vi "Init Device.vi"(8 "error in (no error)":errorcluster, 11 "TE2000 in":refnum<class "Eclipse TI.lvclass">) -> (0 "error out":errorcluster, 3 "TE2000 out":refnum<class "Eclipse TI.lvclass">)   [LabVIEW 2015, in "Eclipse TI.lvlib" / "Eclipse TI.lvclass"]
uses:
  Eclipse TI.lvclass
  Eclipse TI.lvclass/Eclipse TI.ctl
  <vilib>/Instr/_visa.llb/VISA Configure Serial Port (Instr).vi
  Device/Device.lvclass
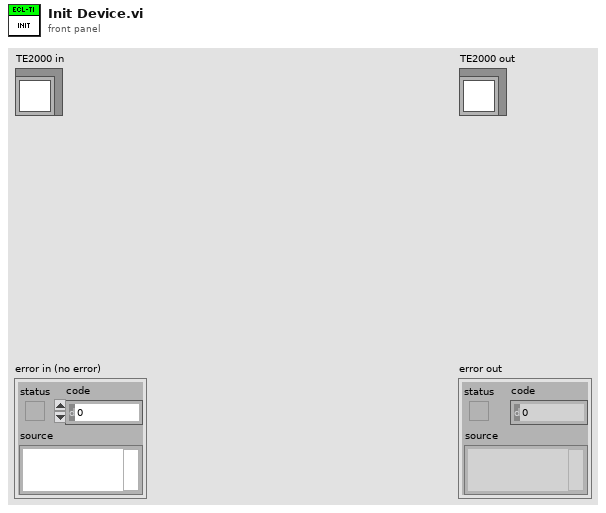
[diagram p1: front panel]
types:
  T1 = typedef "Microscope Type.ctl" = enum16{"TE2000", "Eclipse Ti"}
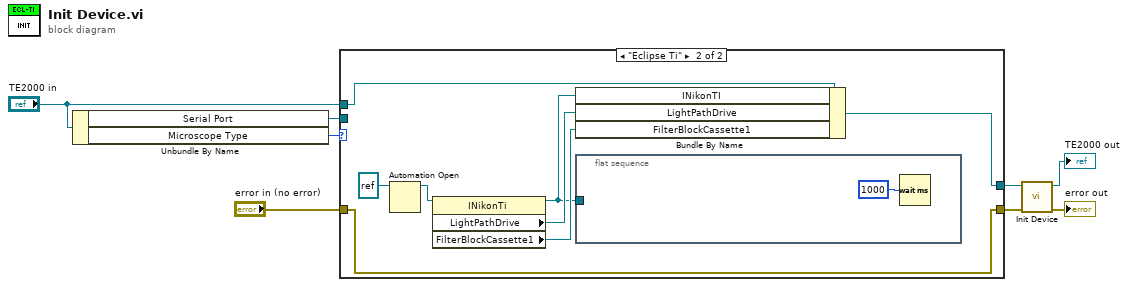
[diagram p0: block diagram]
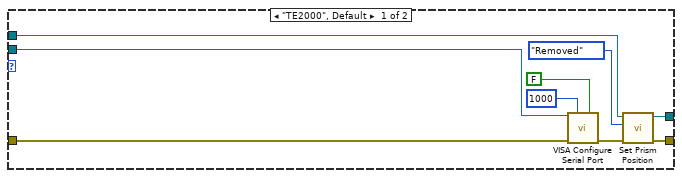
[diagram p2: hidden frame]
diagram:
  n1 = Unbundle By Name("TE2000 in") -> ("Serial Port"=w6:refnum<visa-resource-name>, "Microscope Type"=w1:T1)
  n2 = case shown="\"Eclipse Ti\"" w1 {
    tunnel: w6 -> [w15 _]
    tunnel: "error in (no error)" -> [w14 w18]
    tunnel: "TE2000 in" -> [w13 w23]
    tunnel: [w10 w20] -> w3
    tunnel: [w9 w18] -> w2
    frame "TE2000", Default {
      n3 = call-poly "VISA Configure Serial Port"("VISA resource name"=w15, "timeout (10sec)"=u32 1000, "Enable Termination\nChar (T)"=FALSE ("Enable Termination\nChar (T)"), "error in (no error)"=w14) -> ("error out"=w12:errorcluster)  [unwired: 10 in, 1 out]
      n4 = call-dynamic "Set Prism Position.vi"("error in (no error)"=w12, "Prism Position"=enum16{"Removed", "Inserted"}."Removed", "TE2000 in"=w13) -> ("error out"=w9:errorcluster, "TE2000 out"=w10:refnum<class "Eclipse TI.lvclass">)  [unwired: 7 in]
    }
    frame "Eclipse Ti" {
      n5 = Automation Open(Automation Refnum=refnum<k7> refnum ("TISCOPELib.INikonTi")) -> (Automation Refnum=w24:refnum<k7>)  [unwired: 1 in, 3 out]
      n6 = property class="INikonTi"(reference=w24) -> (reference out=w19:refnum<k7>, "LightPathDrive"=w22:refnum<k7>, "FilterBlockCassette1"=w21:refnum<k7>)  [unwired: 1 in, 1 out]
      n7 = Bundle By Name(cluster=w23, "INikonTI"=w19, "LightPathDrive"=w22, "FilterBlockCassette1"=w21) -> (w20:refnum<class "Eclipse TI.lvclass">)
      n8 = flat-sequence {
        tunnel: w19 -> [_]
        frame #0 {
          n9 = Wait (ms)(milliseconds to wait=u32 1000) -> ()  [unwired: 1 out]
        }
      }
    }
  }
  n10 = call-parent "Init Device.vi"("error in (no error)"=w2, "Device in"=w3) -> ("error out"=→"error out":errorcluster, "Device out"=→"TE2000 out":refnum<class "Eclipse TI.lvclass">)  [unwired: 8 in]
